vi "flow-builder.ec-dosing.vi"(7 "Proc Name":string, 8 "error in":errorcluster, 9 "Unit Index":i32, 11 "Cluster":T3 {"ORP Dosing"."MIX Limit" format="%d [s]"; "ORP Dosing"."MIX Dose" format="%d [s]"; "PH Dosing"."ACID Limit" format="%d [s]"; "PH Dosing"."BASE Limit" format="%d [s]"; "PH Dosing"."ACID Dose" format="%d [s]"; "PH Dosing"."BASE Dose" format="%d [s]"; "EC Dosing"."BETA2 Limit" format="%d [s]"; "EC Dosing"."ALFA2 Limit" format="%d [s]"; "EC Dosing"."ALFA2 Dose" format="%d [s]"; "EC Dosing"."BETA2 Dose" format="%d [s]"; "EC Dosing"."BETA1 Limit" format="%d [s]"; "EC Dosing"."ALFA1 Limit" format="%d [s]"; "EC Dosing"."ALFA1 Dose" format="%d [s]"; "EC Dosing"."BETA1 Dose" format="%d [s]"; "Main"."DailyActivityHours"."Begin Time" format="ON:    %<%H:%M>T"; "Main"."DailyActivityHours"."End Time" format="OFF:    %<%H:%M>T"; "Main"."WashTimes"."Out" format="Wash out: %d [sec]"; "Main"."WashTimes"."In" format="Wash in: %d [sec]"; "Water Dosing"."Water Limit" format="%d [s]"; "Water Dosing"."Water Dose" format="%d [s]"}) -> (0 "error out":errorcluster, 1 "WillDose?":bool, 2 "status":string, 3 "Flow out":T1[](array[typedef]))   [LabVIEW 2024]
uses:
  controls/UiNutritionPanel.ctl
  controls/UiScheduleTimestamp.ctl
  controls/UiStepBuilder.ctl
  controls/type.step-builder.ctl
  controls/enum-ntr-io-format.ctl
  io.interface.serial.vi
  <vilib>/Utility/error.llb/Clear Errors.vi
  <vilib>/Utility/error.llb/Trim Whitespace One-Sided.vi
  globals/globals-engine.vi
  step.util.flag-matching.vi
  util.file.record.vi
  Polymorphics/variantCtrlIo.vi
  util.environment.vi
  util-address-parser.vi
  util-address-builder.vi
  util.DO.ToString.vi
  Polymorphics/io.command-builder.vi
  Polymorphics/io.command-builder.DO.vi
  Polymorphics/io.command-builder.AI.vi
  Polymorphics/io.command-builder.DI.vi
  io.frame.vi
  io.visa.vi
  io.responseValidator.vi
  Polymorphics/io.command-parser.DI.vi
  Polymorphics/io.command-parser.AI.vi
panel:
  out "Dosing Tabel":cluster{"Dose Time":dbl, "Input":string}[](array[cluster])
  out "High Range":bool
  out "Low Range":bool
  out "Low Alarm":bool
  out "High Alarm":bool
  # "Water"
  # "EC"
  # "PH"
  # "ORP"
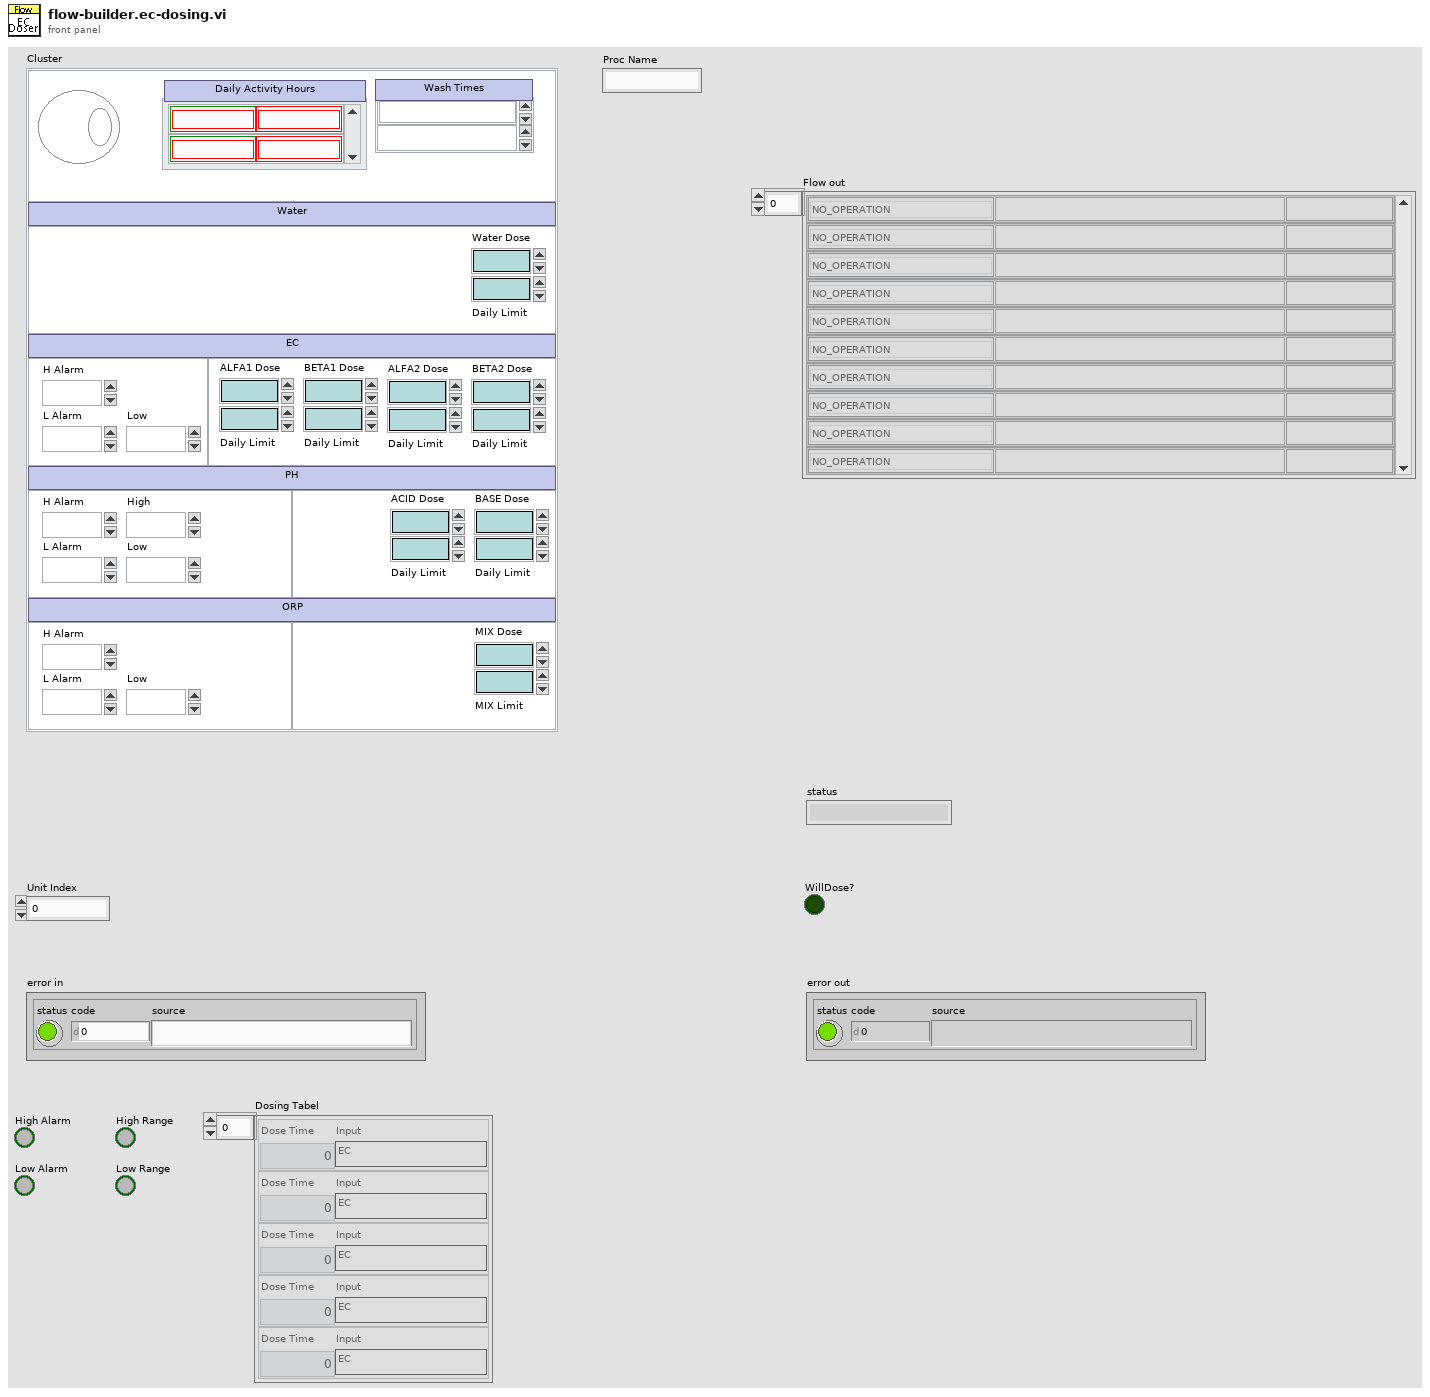
[diagram p1: front panel]
types:
  T1 = typedef "UiStepBuilder.ctl" = cluster{"Step Function":T2, "ParamString":string, "Step Label":string}
  T2 = typedef "type.step-builder.ctl" = enum16{"NO_OPERATION", "DELAY-JUMP", "DELAY", "JUMP", "COMPLETE", "SCHEDULER", "IRR-CHECK", "UNIT-CHECK", "UNIT-SAMPLE", "UNIT-DOSE", "LOG-REPORT", "LOG-MESSAGE", "IO-READ", "IO-READ-MANY", "IO-WRITE", "IO-COMPARE-OUT", "IO-COMPARE-IN", "PROC-START", "PROC-STOP", "PROC-LOAD", "PROC-IS-COMPLETED", "RECORD-MOVE", "GET-RH", "GET-UV", "GET-WD", "GET-WS", "OCS-CHECK", "OCS-RECORD"}
  T3 = typedef "UiNutritionPanel.ctl" = cluster{"Main":cluster{"Enable":bool, "WashTimes":cluster{"In":dbl, "Out":dbl}, "DailyActivityHours":cluster{"Begin Time":T4, "End Time":T4}[]}, "Water Dosing":cluster{"Water Dose":dbl, "Water Limit":dbl}, "EC Ranges":cluster{"H Alarm":dbl, "L Alarm":dbl, "Low":dbl}, "EC Dosing":cluster{"ALFA1 Dose":dbl, "ALFA1 Limit":dbl, "BETA1 Dose":dbl, "BETA1 Limit":dbl, "ALFA2 Dose":dbl, "ALFA2 Limit":dbl, "BETA2 Dose":dbl, "BETA2 Limit":dbl}, "PH Ranges":cluster{"H Alarm":dbl, "L Alarm":dbl, "High":dbl, "Low":dbl}, "PH Dosing":cluster{"ACID Dose":dbl, "ACID Limit":dbl, "BASE Dose":dbl, "BASE Limit":dbl}, "ORP Ranges":cluster{"H Alarm":dbl, "L Alarm":dbl, "Low":dbl}, "ORP Dosing":cluster{"MIX Dose":dbl, "MIX Limit":dbl}}
  T4 = typedef "UiScheduleTimestamp.ctl" = timestamp
  T5 = typedef "enum-ntr-io-format.ctl" = enum16{"UN_VLV%d", "UN_PMP%d", "UN_WL%d", "UN_PH", "UN_EC", "UN_ORP", "UN_WT", "UN_PH2", "UN_ALFA1", "UN_BETA1", "UN_ALFA2", "UN_BETA2", "UN_ACID", "UN_BASE", "UN_WATER", "UN_ORPMIX"}
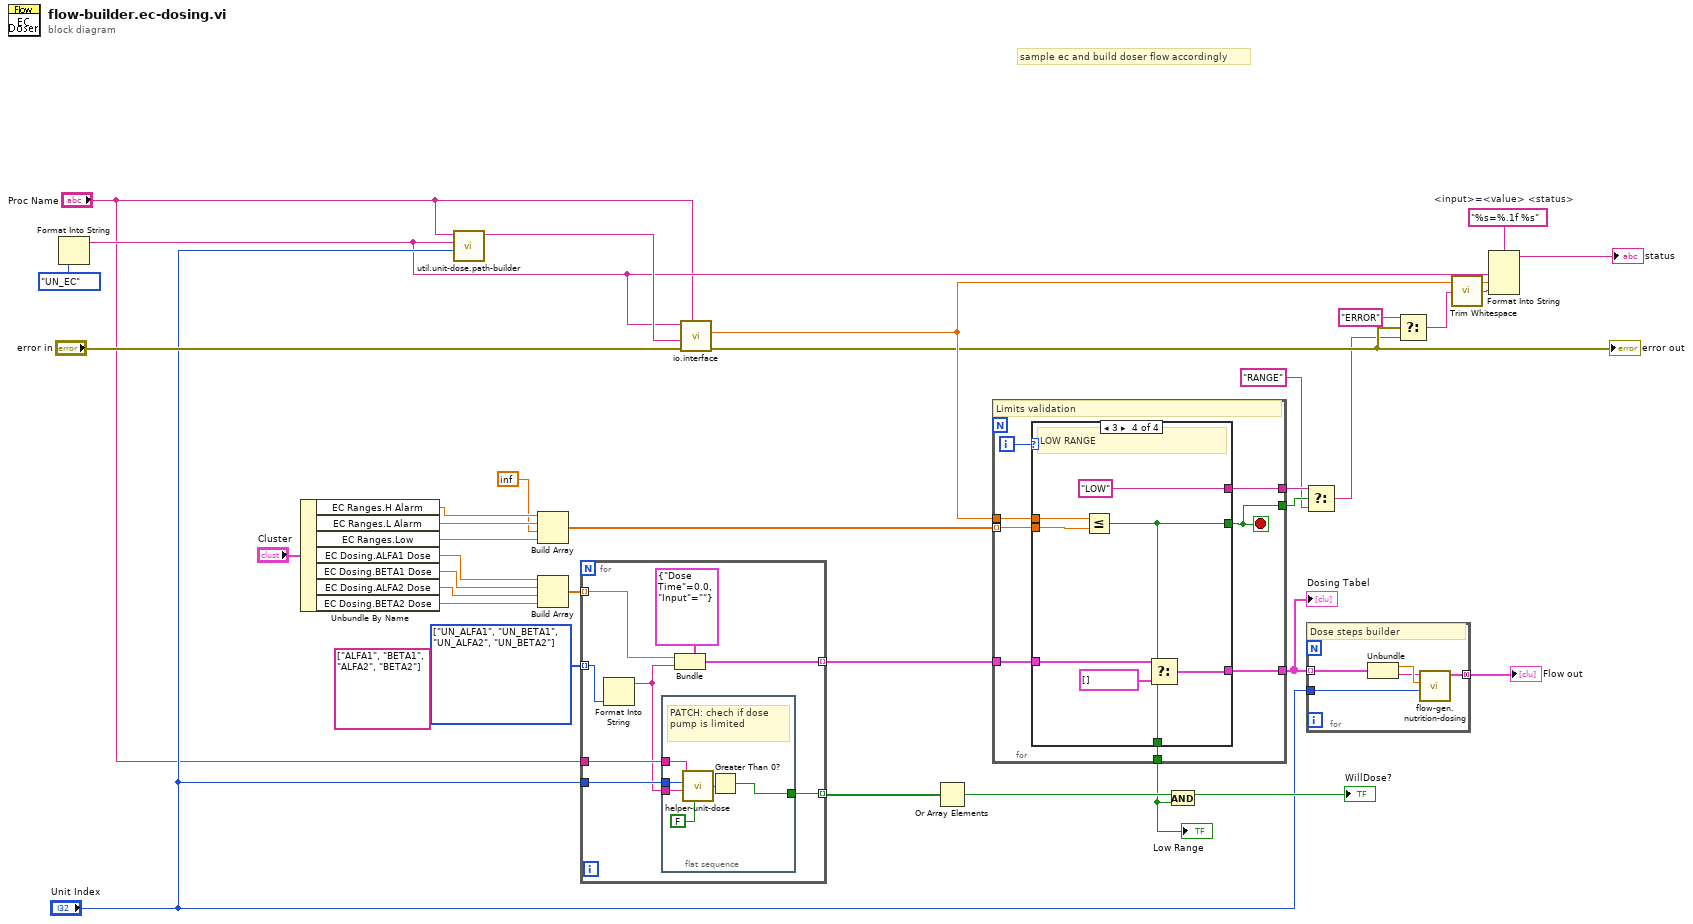
[diagram p0: block diagram]
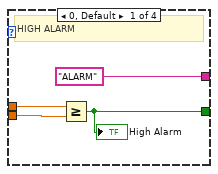
[diagram p2: hidden frame]
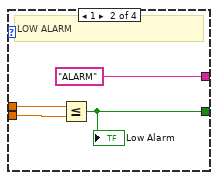
[diagram p3: hidden frame]
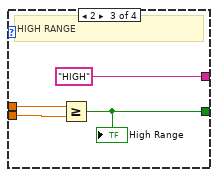
[diagram p4: hidden frame]
diagram:
  (unwired) string[] ["ALFA1", "BETA1", "ALFA2", "BETA2"] ("I/O")
  w17 = "%s=%.1f %s"  # <input>=<value> <status>
  w23 = T5[] [enum."UN_ALFA1", enum."UN_BETA1", enum."UN_ALFA2", enum."UN_BETA2"] items=["UN_VLV%d", "UN_PMP%d", "UN_WL%d", "UN_PH", "UN_EC", "UN_ORP", "UN_WT", "UN_PH2", "UN_ALFA1", "UN_BETA1", "UN_ALFA2", "UN_BETA2", "UN_ACID", "UN_BASE", "UN_WATER", "UN_ORPMIX"] ("I/O")
  # "sample ec and build doser flow accordingly"
  n1 = Format Into String(enum-ntr-io-format."UN_EC") -> (resulting string=w2:string)  [unwired: 3 in, 1 out]
  n2 = Unbundle By Name("Cluster") -> ("EC Ranges.H Alarm"=w36:dbl, "EC Ranges.L Alarm"=w31:dbl, "EC Ranges.Low"=w19:dbl, "EC Dosing.ALFA1 Dose"=w29:dbl, "EC Dosing.BETA1 Dose"=w28:dbl, "EC Dosing.ALFA2 Dose"=w27:dbl, "EC Dosing.BETA2 Dose"=w26:dbl)
  n3 = call "util.unit-dose.path-builder.vi"("Unit Index"="Unit Index", "Input"=w2, "Proc Name"="Proc Name") -> ("\\NUTRITION\\ORP\\ORP_U1_2024-08-16.*"=w9:string)  [unwired: 8 in]
  n4 = Build Array(w36, w31, inf, w19) -> (w35:dbl[])
  n5 = Build Array(w29, w28, w27, w26) -> (w25:dbl[])
  n6 = for {
    tunnel: w25 -> [w44] mode=indexing
    tunnel: [w43] -> w24 mode=indexing
    tunnel: w23 -> [w38] mode=indexing
    tunnel: "Proc Name" -> [w41]
    tunnel: "Unit Index" -> [w40]
    tunnel: [w39] -> w14 mode=indexing
    n7 = Format Into String(w38) -> (resulting string=w37:string)  [unwired: 3 in, 1 out]
    n8 = flat-sequence {
      tunnel: w40 -> [w50]
      tunnel: [w48] -> w39
      tunnel: w41 -> [w46]
      tunnel: w37 -> [w45]
      frame #0 {
        # "PATCH: chech if dose pump is limited"
        n9 = call "helper-unit-dose.vi"("Auto Update Limit Record? (T)"=FALSE ("(F)ReadOnly/(T)Auto Update"), "output"=w45, "Unit Index"=w50, "Proc Name"=w46) -> ("Actual Dose in Seconds"=w49:i32)  [unwired: 5 in, 2 out]
        n10 = Greater Than 0?(x=w49) -> (x > 0?=w48:bool)
      }
    }
    n11 = Bundle(cluster=cluster{"Dose Time":dbl, "Input":string} {"Dose Time"=0.0, "Input"=""} ("Cluster"), "Dose Time"=w44, "Input"=w37) -> (w43:cluster{"Dose Time":dbl, "Input":string})
  }
  n12 = call "io.interface.vi"("Caller"="Proc Name", "error in"="error in", "record filename.* (disabled if empty)"=w9, "IO Name in"=w2) -> ("error out"=w7:errorcluster, "Value out"=w16:dbl)  [unwired: 2 in, 4 out]
  "error out" <- w7
  n13 = Or Array Elements(Boolean array=w14) -> (logical OR=w13:bool)
  n14 = for {
    tunnel: w35 -> [w57] mode=indexing
    tunnel: [w56] -> w33
    tunnel: w16 -> [w55]
    tunnel: [w54] -> w34
    tunnel: w24 -> [w53]
    tunnel: [w52] -> w22
    tunnel: [w51] -> w11
    i -> [w58]
    stop <- w54 stop-if-true
    # "Limits validation"
    n15 = case shown="3" w58 {
      tunnel: w57 -> [w61 w65 w69 w76]
      tunnel: [w59 w63 w67 w71] -> w54
      tunnel: ["ALARM" "ALARM" "HIGH" "LOW"] -> w56
      tunnel: w55 -> [w60 w64 w68 w75]
      tunnel: [_ _ _ w74] -> w52
      tunnel: w53 -> [_ _ _ w73]
      tunnel: [_ _ _ w71] -> w51
      frame 0, Default {
        # "HIGH ALARM"
        n16 = Greater Or Equal?(x=w60, y=w61) -> (x >= y?=w59:bool)
        "High Alarm" <- w59
      }
      frame 1 {
        # "LOW ALARM"
        n17 = Less Or Equal?(x=w64, y=w65) -> (x <= y?=w63:bool)
        "Low Alarm" <- w63
      }
      frame 2 {
        # "HIGH RANGE"
        n18 = Greater Or Equal?(x=w68, y=w69) -> (x >= y?=w67:bool)
        "High Range" <- w67
      }
      frame 3 {
        # "LOW RANGE"
        n19 = Less Or Equal?(x=w75, y=w76) -> (x <= y?=w71:bool)
        n20 = Select(t=w73, s=w71, f=cluster{"BETA-2":dbl, "I/O":string}[] []) -> (s? t:f=w74:cluster{"BETA-2":dbl, "I/O":string}[])
      }
    }
  }
  "Dosing Tabel" <- w22
  "Low Range" <- w11
  n21 = And(x=w13, y=w11) -> (x .and. y?=→"WillDose?":bool)
  n22 = Select(t=w33, s=w34, f="RANGE") -> (s? t:f=w6:string)
  n23 = for {
    tunnel: [w82] -> w21 mode=concatenating
    tunnel: w22 -> [w81] mode=indexing
    tunnel: "Unit Index" -> [w78]
    # "Dose steps builder"
    n24 = Unbundle(w81) -> ("BETA-2"=w80:dbl, "I/O"=w79:string)
    n25 = call "flow-gen.nutrition-dosing.vi"("Unit Index"=w78, "Dosing Time"=w80, "IO Name"=w79) -> ("Flow"=w82:T1[])  [unwired: 7 in, 1 out]
  }
  "Flow out" <- w21
  n26 = Select(t="ERROR", s=w7, f=w6) -> (s? t:f=w5:string)
  n27 = call <vilib>:"Trim Whitespace.vi"("string"=w5) -> ("trimmed string"=w8:string)  [unwired: 1 in]
  n28 = Format Into String(format string=w17, w2, w16, w8) -> (resulting string=→"status":string)  [unwired: 2 in, 1 out]
